vi "Arduino Stepper Driver XY subVI gotoPos.vi"(8 "error in (no error)":errorcluster, 9 "Vertical Set Position":i32, 10 "Horizontal Set Position":i32, 11 "VISA resource name":refnum<visa-resource-name>) -> (0 "error out":errorcluster, 3 "VISA resource name out":refnum<visa-resource-name>)   [LabVIEW 2013]
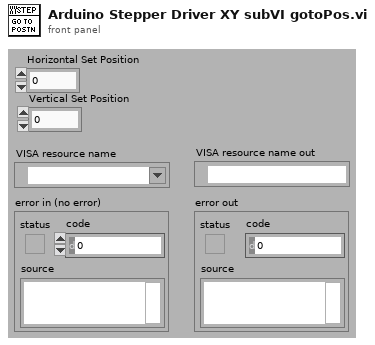
[diagram p1: front panel]
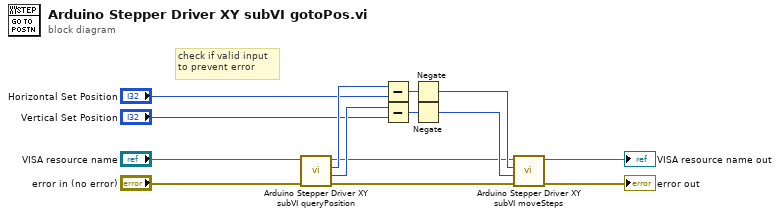
[diagram p0: block diagram]
diagram:
  # "check if valid input\nto prevent error"
  n1 = call "Arduino Stepper Driver XY subVI queryPosition.vi"("error in (no error)"="error in (no error)", "VISA resource name"="VISA resource name") -> ("error out"=w2:errorcluster, "Vertical driver position"=w11:i32, "Horizontal driver position"=w12:i32, "VISA resource name out"=w1:refnum<visa-resource-name>)  [unwired: 6 in]
  n2 = Subtract(x=w12, y="Horizontal Set Position") -> (x-y=w8:i32)
  n3 = Subtract(x=w11, y="Vertical Set Position") -> (x-y=w6:i32)
  n4 = Negate(x=w8) -> (-x=w7:i32)
  n5 = Negate(x=w6) -> (-x=w5:i32)
  n6 = call "Arduino Stepper Driver XY subVI moveSteps.vi"("error in (no error)"=w2, "input steps V"=w5, "input steps H"=w7, "VISA resource name"=w1) -> ("error out"=→"error out":errorcluster, "VISA resource name out"=→"VISA resource name out":refnum<visa-resource-name>)  [unwired: 6 in]
